vi "ROE200_VisaInit_debugREP.vi"(8 "error in (no error)":errorcluster, 11 "VISA resource name":refnum<visa-resource-name>) -> (0 "error out":errorcluster, 3 "VISA resource name out":refnum<visa-resource-name>, 4 "error in initialization":bool)   [LabVIEW 2015]
panel:
  out "appended array":u32[](array[numeric])
  out "Active Drive":u8
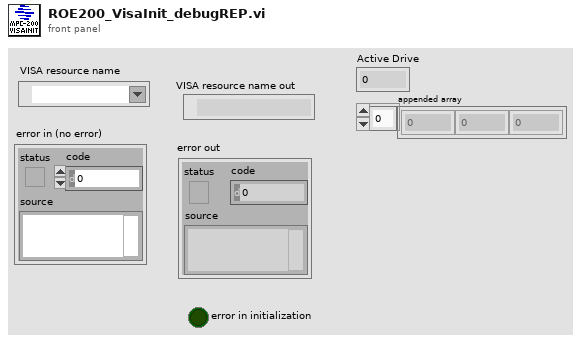
[diagram p1: front panel]
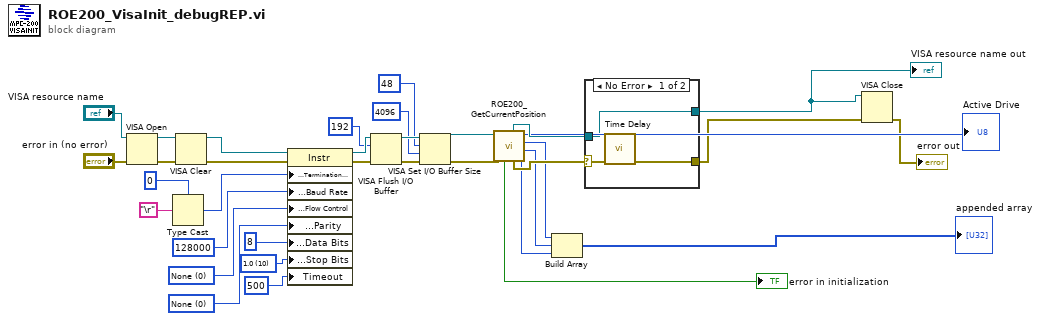
[diagram p0: block diagram]
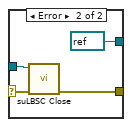
[diagram p2: hidden frame]
diagram:
  w20 = u16 10 items=["1.0"=10, "1.5"=15, "2.0"=20] ("Serial Settings:Serial Stop Bits")
  w21 = u16 0 items=["None", "Odd", "Even", "Mark", "Space"] ("Serial Settings:Serial Parity")
  w23 = u16 0 items=["None", "XON/XOFF", "RTS/CTS", "XON/XOFF & RTS/CTS", "DTR/DSR", "XON/XOFF & DTR/DSR"] ("Serial Settings:Serial Flow Control")
  n1 = VISA Open(error in (no error)="error in (no error)", VISA resource name="VISA resource name") -> (VISA resource name=w35:refnum<visa-resource-name>, error out=w34:errorcluster)  [unwired: 3 in]
  n2 = Type Cast(type=u8 0, x="\r") -> (*(type *) &x=w25:u8)
  n3 = VISA Clear(VISA resource name=w35, error in (no error)=w34) -> (VISA resource name out=w16:refnum<visa-resource-name>, error out=w15:errorcluster)
  n4 = property class="Instr"(reference=w16, error in=w15, "Message Based Settings:Termination Character"=w25, "Serial Settings:Baud Rate"=u32 128000 ("Serial Settings:Serial Baud Rate"), "Serial Settings:Flow Control"=w23, "Serial Settings:Parity"=w21, "Serial Settings:Data Bits"=u16 8 ("Serial Settings:Serial Data Bits"), "Serial Settings:Stop Bits"=w20, "Timeout"=u32 500 ("General Settings:Timeout Value")) -> (reference out=w30:refnum<visa-resource-name>, error out=w32:errorcluster)
  n5 = VISA Flush I/O Buffer(VISA resource name=w30, mask (16)=u16 192, error in (no error)=w32) -> (VISA resource name out=w33:refnum<visa-resource-name>, error out=w31:errorcluster)
  n6 = VISA Set I/O Buffer Size(VISA resource name=w33, mask (16)=u16 48, size (4096)=u32 4096 ("size (0)"), error in (no error)=w31) -> (VISA resource name out=w14:refnum<visa-resource-name>, error out=w13:errorcluster)
  n7 = call "ROE200_GetCurrentPosition.vi"("error in (no error)"=w13, "VISA resource name"=w14) -> ("Z Position"=w6:u32, "Y Position"=w7:u32, "X Position"=w8:u32, "Active Drive"=→"Active Drive":u8, "error out"=w11:errorcluster, "VISA resource  out"=w12:refnum<visa-resource-name>, "error in GetCurrentPosition"=→"error in initialization":bool)  [unwired: 3 in]
  n8 = Build Array(w8, w7, w6) -> (→"appended array":u32[])
  n9 = case shown="No Error" w11 {
    selector: w11 -> [w36 w40]
    tunnel: w12 -> [w38 w41]
    tunnel: [w38 refnum<visa-resource-name> refnum ("VISA resource name out")] -> w3
    tunnel: [w37 w42] -> w2
    frame No Error {
      n10 = call "Time Delay"("error in (no error)"=w36) -> ("error out"=w37:errorcluster)  [unwired: 10 in]
    }
    frame Error {
      n11 = call "suLBSC Close.vi"("error in (no error)"=w40, "VISA resource name"=w41) -> ("error out"=w42:errorcluster)  [unwired: 9 in]
    }
  }
  "VISA resource name out" <- w3
  n12 = VISA Close(VISA resource name=w3, error in (no error)=w2) -> (error out=→"error out":errorcluster)
